vi "Machine Id Selection.vi"() -> (2 "Action":bool)   [LabVIEW 2015]
uses:
  Machine id selection.ctl
  Feature list/Control PB/Next_.ctl
  Galobal variable_TI.vi
panel:
  out "Boolean":bool
  in  "Next":T1
  in  "Exit":bool
  in  "Machine Name":T2
  out "element":string
  out "ID Data":cluster{"Array":string[][]}
  # "Machine Name"
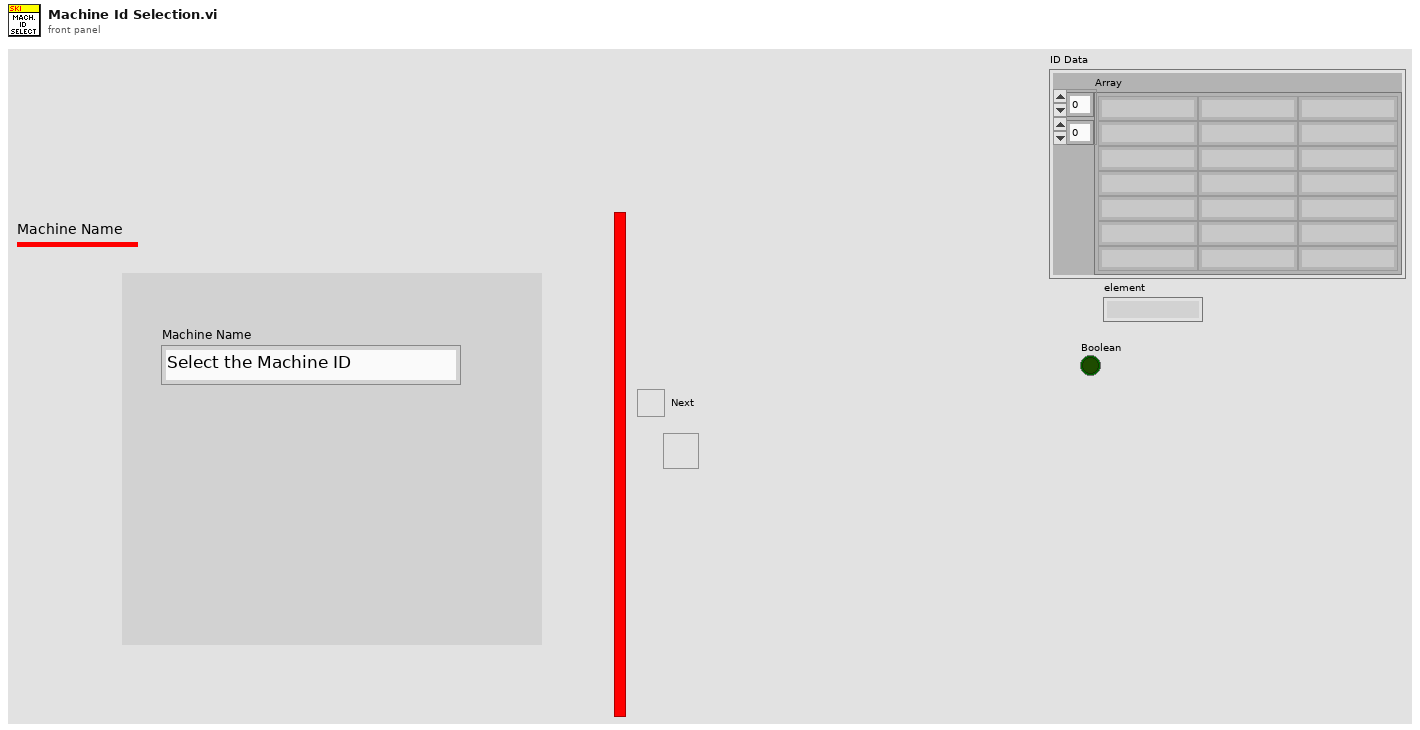
[diagram p1: front panel]
types:
  T1 = typedef "Next_.ctl" = bool
  T2 = typedef "Machine id selection.ctl" = enum16{"Select the Machine ID", "YCA", "YHB", "YSD", "Job_Id-62"}
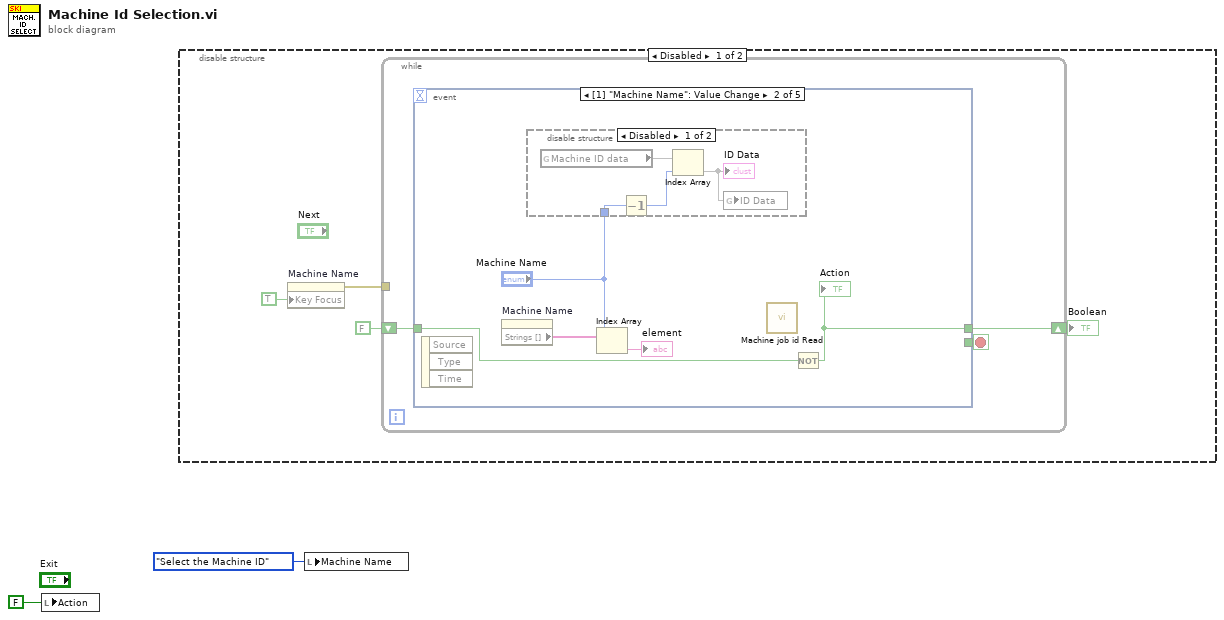
[diagram p0: block diagram]
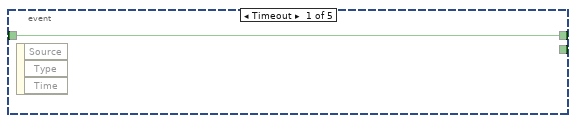
[diagram p2: hidden frame]
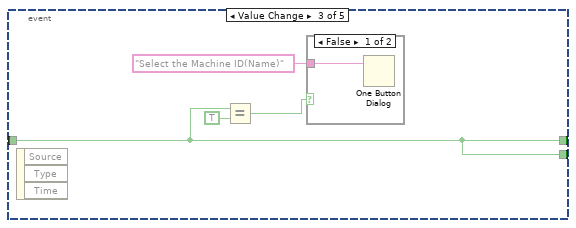
[diagram p4: hidden frame]
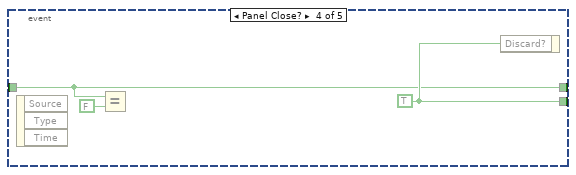
[diagram p6: hidden frame]
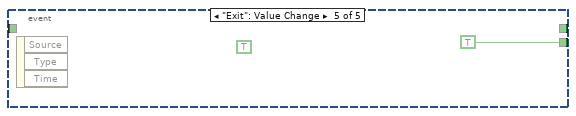
[diagram p7: hidden frame]
diagram:
  n1 = local write "Action"(FALSE ("Boolean 2")) -> ()
  n2 = disable-structure shown="Disabled" {
    frame Disabled {
      n3 = property on="Machine Name" class="Enum (strict)"("Key Focus"=TRUE) -> (error out=w4:errorcluster)  [unwired: 2 in, 1 out]
      n4 = while {
        shift-right: [w8] -> w3
        shift-left: FALSE -> [w7]
        tunnel: w4 -> [_]
        stop <- w9 stop-if-true
        n5 = event shown="[1] \"Machine Name\": Value Change" {
          selector: _ -> [_ _ _ _ _]
          dyn-events: _ -> [_ _ _ _ _]
          timeout: _ -> [_ _ _ _ _]
          tunnel: [_ _ w22 w27 TRUE ("Discard?")] -> w9
          tunnel: [w10 w12 w22 w26 _] -> w8
          tunnel: w7 -> [w10 w15 w22 w26 _]
          event Timeout {
            n6 = event-data() -> ()  [unwired: 1 in, 3 out]
          }
          event Value Change {
            n7 = event-data() -> ()  [unwired: 1 in, 3 out]
            n8 = property on="Machine Name" class="Enum (strict)"() -> ("Strings []"=w14:string[])  [unwired: 2 in, 2 out]
            n9 = disable-structure shown="Disabled" {
              disable-tunnel: "Machine Name" -> [w17 _]
              frame Disabled {
                n10 = global read "Galobal variable_TI.vi" "Machine ID data"() -> (w19)
                n11 = Decrement(x=w17) -> (x-1=w16:T2)
                n12 = Index Array(array=w19, index=w16) -> (element=w18)
                "ID Data" <- w18
                n13 = global write "Galobal variable_TI.vi" "ID Data"(w18) -> ()
              }
              frame Enabled {
              }
            }
            n14 = Index Array(array=w14, index="Machine Name") -> (element=→"element":string)
            n15 = call "Machine job id Read.vi"() -> ()  [unwired: 11 in, 1 out]
            n16 = Not(x=w15) -> (.not. x?=w12:bool)
            "Action" <- w12
          }
          event Value Change {
            n17 = event-data() -> ()  [unwired: 1 in, 3 out]
            n18 = Equal?(x=w22, y=TRUE) -> (x = y?=w20:bool)
            n19 = case shown="False" w20 {
              tunnel: "Select the Machine ID(Name)" -> [w24 _]
              frame False {
                n20 = One Button Dialog(message=w24) -> ()  [unwired: 1 in, 1 out]
              }
              frame True {
              }
            }
          }
          event Panel Close? {
            w27 = TRUE ("Discard?")
            n21 = event-data() -> ()  [unwired: 1 in, 3 out]
            n22 = Equal?(x=w26, y=FALSE) -> ()  [unwired: 1 out]
            n23 = event-data("Discard?"=w27) -> ()  [unwired: 1 in, 1 out]
          }
          event "Exit": Value Change {
            (unwired) TRUE ("y")
            n24 = event-data() -> ()  [unwired: 1 in, 3 out]
          }
        }
      }
      "Boolean" <- w3
    }
    frame Enabled {
    }
  }
  n25 = local write "Machine Name"(Machine_id_selection."Select the Machine ID" ("Machine Name")) -> ()
